vi "buma.vi"(11 "Numeric":i32) -> (3 "String":string)   [LabVIEW 2022 SP3]
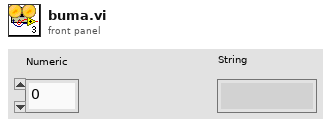
[diagram p1: front panel]
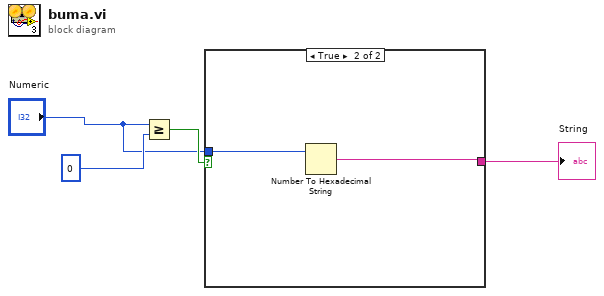
[diagram p0: block diagram]
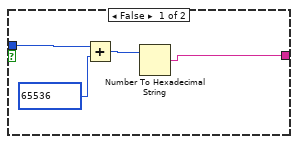
[diagram p2: hidden frame]
diagram:
  n1 = Greater Or Equal?(x="Numeric", y=0) -> (x >= y?=w3:bool)
  n2 = case shown="True" w3 {
    tunnel: "Numeric" -> [w7 w10]
    tunnel: [w5 w9] -> w1
    frame False {
      n3 = Add(x=w7, y=65536) -> (x+y=w6:i32)
      n4 = Number To Hexadecimal String(2:w6) -> (0:w5:string)  [unwired: 1 in]
    }
    frame True {
      n5 = Number To Hexadecimal String(2:w10) -> (0:w9:string)  [unwired: 1 in]
    }
  }
  "String" <- w1
